vi "2Darray2DDT.vi"(3 "rate":dbl, 4 "StartTime":timestamp, 5 "2D Array":dbl[][](array[numeric])) -> (1 "Dynamic Data Type":dynamicdata(graph), 2 "EndTime":timestamp)   [LabVIEW 2015]
uses:
  Instance           1 19Saved   2Darray2DDT .vi
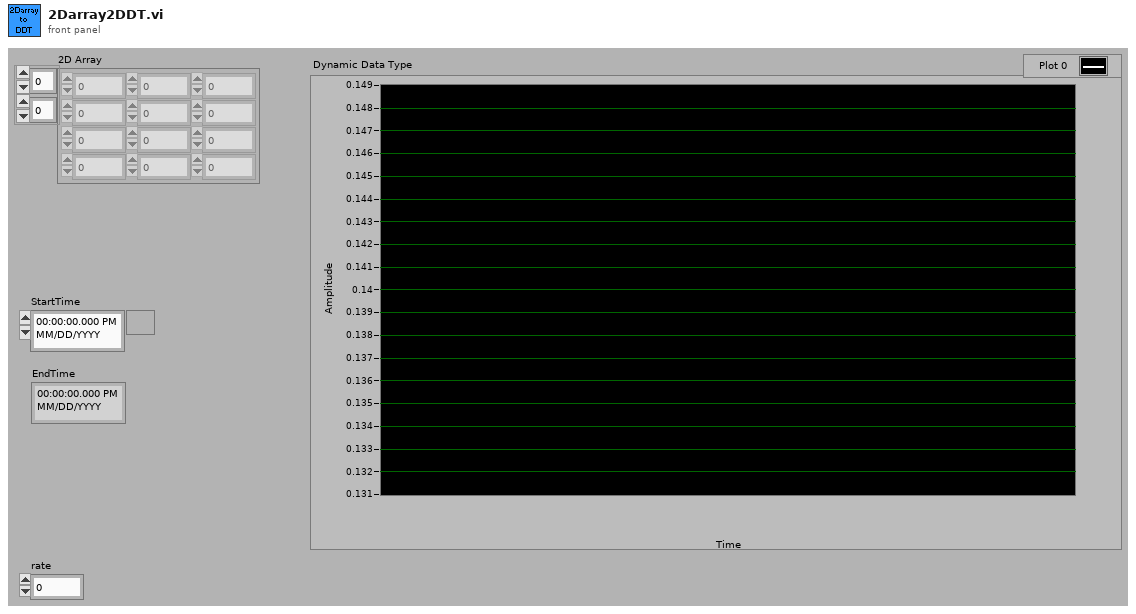
[diagram p1: front panel]
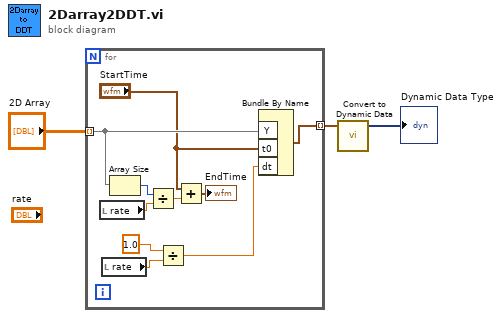
[diagram p0: block diagram]
diagram:
  n1 = for {
    tunnel: "2D Array" -> [w11] mode=indexing
    tunnel: [w13] -> w1 mode=indexing
    n2 = local read "rate"() -> (w8:dbl)
    n3 = local read "rate"() -> (w10:dbl)
    n4 = Array Size(array=w11) -> (size(s)=w9:i32)
    n5 = Divide(x=w9, y=w8) -> (x/y=w6:dbl)
    n6 = Divide(x=1.0, y=w10) -> (x/y=w7:dbl)
    n7 = Add(x="StartTime", y=w6) -> (x+y=→"EndTime":timestamp)
    n8 = Bundle By Name("Y"=w11, "t0"="StartTime", "dt"=w7) -> (w13:waveform(dbl))  [unwired: 1 out]
  }
  n9 = call "Convert to Dynamic Data"("Array of Waveforms"=w1) -> ("Dynamic Data Type"=→"Dynamic Data Type":dynamicdata)  [unwired: 3 out]
